vi "MGI Edge Enhance 2D Array.vi"(1 "Array[][]":sgl[][](array[numeric]) format="%.2f") -> (0 "Smoothed Array[][]":sgl[][](array[numeric]) format="%.2f")   [LabVIEW 2020]
doc: "Perform an edge enhancement operation on a 2D array based on the absolute value of differences between neighbors of a point in opposite directions. It doesn't sharpen edges, but it does damp out constant regions.\n\nAuthored by David A. Moore\nsupport@mooregoodideas.com\nwww.mooregoodideas.com\n\nCopyright (c) 2010, Moore Good Ideas, Inc.\n\nAll rights reserved.\n\nRedistribution and use in source and binary forms, with or without modification, are permitted provided that the following conditions are met:\n\n * Redistributions of source code must retain the above copyright notice, this list of conditions and the following disclaimer.\n * Redistributions in binary form must reproduce the above copyright notice, this list of conditions and the following disclaimer in the documentation and/or other materials provided with the distribution.\n * Neither the name of Moore Good Ideas, Inc. nor the names of its contributors may be used to endorse or promote products derived from this software without specific prior written permission.\n\nTHIS SOFTWARE IS PROVIDED BY THE COPYRIGHT HOLDERS AND CONTRIBUTORS \"AS IS\" AND ANY EXPRESS OR IMPLIED WARRANTIES, INCLUDING, BUT NOT LIMITED TO, THE IMPLIED WARRANTIES OF MERCHANTABILITY AND FITNESS FOR A PARTICULAR PURPOSE ARE DISCLAIMED. IN NO EVENT SHALL THE COPYRIGHT OWNER OR CONTRIBUTORS BE LIABLE FOR ANY DIRECT, INDIRECT, INCIDENTAL, SPECIAL, EXEMPLARY, OR CONSEQUENTIAL DAMAGES (INCLUDING, BUT NOT LIMITED TO, PROCUREMENT OF SUBSTITUTE GOODS OR SERVICES; LOSS OF USE, DATA, OR PROFITS; OR BUSINESS INTERRUPTION) HOWEVER CAUSED AND ON ANY THEORY OF LIABILITY, WHETHER IN CONTRACT, STRICT LIABILITY, OR TORT (INCLUDING NEGLIGENCE OR OTHERWISE) ARISING IN ANY WAY OUT OF THE USE OF THIS SOFTWARE, EVEN IF ADVISED OF THE POSSIBILITY OF SUCH DAMAGE."
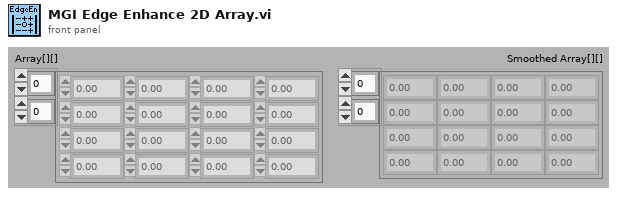
[diagram p1: front panel]
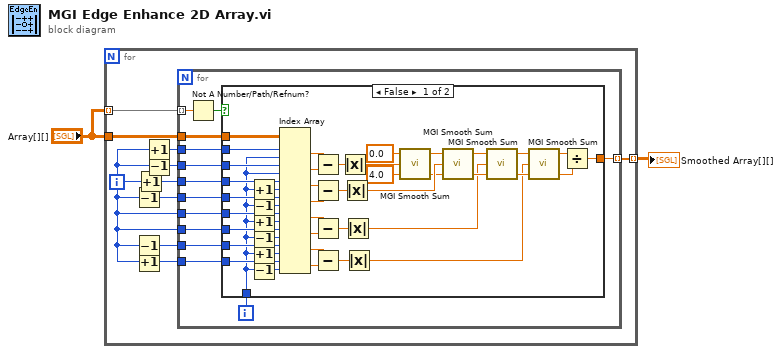
[diagram p0: block diagram]
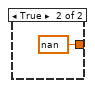
[diagram p2: hidden frame]
diagram:
  n1 = for {
    tunnel: "Array[][]" -> [w12]
    tunnel: "Array[][]" -> [w4] mode=indexing
    tunnel: [w3] -> w1 mode=indexing
    i -> [w9]
    n2 = Decrement(x=w9) -> (x-1=w7:i32)
    n3 = Decrement(x=w9) -> (x-1=w6:i32)
    n4 = Increment(x=w9) -> (x+1=w5:i32)
    n5 = Increment(x=w9) -> (x+1=w8:i32)
    n6 = Increment(x=w9) -> (x+1=w11:i32)
    n7 = Decrement(x=w9) -> (x-1=w10:i32)
    n8 = for {
      tunnel: w12 -> [w25]
      tunnel: w8 -> [w22]
      tunnel: w11 -> [w24]
      tunnel: w10 -> [w23]
      tunnel: w7 -> [w21]
      tunnel: w9 -> [w20]
      tunnel: w9 -> [w19]
      tunnel: w6 -> [w18]
      tunnel: w5 -> [w17]
      tunnel: w4 -> [w14] mode=indexing
      tunnel: [w15] -> w3 mode=indexing
      i -> [w16]
      n9 = Not A Number/Path/Refnum?(number/path/refnum=w14) -> (NaN/Path/Refnum?=w13:bool)
      n10 = case shown="False" w13 {
        tunnel: w25 -> [w68 _]
        tunnel: w24 -> [w67 _]
        tunnel: w23 -> [w66 _]
        tunnel: w22 -> [w65 _]
        tunnel: w21 -> [w64 _]
        tunnel: w20 -> [w63 _]
        tunnel: w19 -> [w62 _]
        tunnel: w18 -> [w61 _]
        tunnel: w17 -> [w60 _]
        tunnel: w16 -> [w59 _]
        tunnel: [w40 sgl nan] -> w15
        frame False {
          n11 = Increment(x=w59) -> (x+1=w55:i32)
          n12 = Decrement(x=w59) -> (x-1=w54:i32)
          n13 = Increment(x=w59) -> (x+1=w50:i32)
          n14 = Decrement(x=w59) -> (x-1=w49:i32)
          n15 = Increment(x=w59) -> (x+1=w45:i32)
          n16 = Decrement(x=w59) -> (x-1=w44:i32)
          n17 = Index Array(array=w68, index (row) #1=w67, index (col) #1=w59, index (row) #2=w66, index (col) #2=w59, index (row) #3=w65, index (col) #3=w55, index (row) #4=w64, index (col) #4=w54, index (row) #5=w63, index (col) #5=w50, index (row) #6=w62, index (col) #6=w49, index (row) #7=w61, index (col) #7=w45, index (row) #8=w60, index (col) #8=w44) -> (element #1=w57:sgl, element #2=w58:sgl, element #3=w53:sgl, element #4=w52:sgl, element #5=w47:sgl, element #6=w48:sgl, element #7=w42:sgl, element #8=w43:sgl)
          n18 = Subtract(x=w57, y=w58) -> (x-y=w56:sgl)
          n19 = Subtract(x=w53, y=w52) -> (x-y=w51:sgl)
          n20 = Subtract(x=w47, y=w48) -> (x-y=w46:sgl)
          n21 = Subtract(x=w42, y=w43) -> (x-y=w41:sgl)
          n22 = Absolute Value(x=w56) -> (abs(x)=w39:sgl)
          n23 = Absolute Value(x=w51) -> (abs(x)=w29:sgl)
          n24 = Absolute Value(x=w46) -> (abs(x)=w26:sgl)
          n25 = Absolute Value(x=w41) -> (abs(x)=w34:sgl)
          n26 = call <userlib>:"MGI Smooth Sum.vi"("Count In"=sgl 4.0, "New Value"=w39, "Sum In"=sgl 0.0) -> ("Count Out"=w28:sgl, "Sum Out"=w30:sgl)  [unwired: 1 in]
          n27 = call <userlib>:"MGI Smooth Sum.vi"("Count In"=w28, "New Value"=w29, "Sum In"=w30) -> ("Count Out"=w27:sgl, "Sum Out"=w31:sgl)  [unwired: 1 in]
          n28 = call <userlib>:"MGI Smooth Sum.vi"("Count In"=w27, "New Value"=w26, "Sum In"=w31) -> ("Count Out"=w36:sgl, "Sum Out"=w35:sgl)  [unwired: 1 in]
          n29 = call <userlib>:"MGI Smooth Sum.vi"("Count In"=w36, "New Value"=w34, "Sum In"=w35) -> ("Count Out"=w32:sgl, "Sum Out"=w33:sgl)  [unwired: 1 in]
          n30 = Divide(x=w33, y=w32) -> (x/y=w40:sgl)
        }
        frame True {
        }
      }
    }
  }
  "Smoothed Array[][]" <- w1
